vi "NFindBlock.vi"(6 "Start pos":dbl[](array[numeric])=[1161.9163378402552, 774.3453732417895, -2809.9800957108705], 7 "Robot pos":dbl[](array[numeric])=[1630.1539120368434, 560.2708584885918, -4533.599258498874], 9 "Y array":dbl[](array[numeric])=[1951.9460733978328, 2174.013680158977, 2100.374349178618, 2027.3757209543814, 1956.3808654729685, 1887.0818616789568, 1760.9212330614585, 1711.1248280430027, 1665.8553251480664, 1620.1460768722577, 1574.622711636553, 1528.915202610297, 1482.2464785728923, 1343.483778512897, 1271.9279899122423, 1200.9260176050532, 1130.2822245353427, 1056.6497434670005, 977.0249347379225, 894.9824777519775, 813.45928692706, 728.5434146890511, 639.3942546253647, 549.8327407334499, 1303.2154100813484, 1326.243227689847, 1344.7706940544083, 1355.2988665944963, 1366.388334703981, 1376.2633344507678, 1387.3858605477956, 1387.3395311652666, 1396.1291038661302, 1403.8469963592477, 1406.044876812333, 1415.0186919401144, 1397.8349011686557, 1389.429356203805, 1373.0493553890178, 1358.50073650405, 1336.518228027625, 1318.298945741701, 1298.2767133270827, 1269.645856509089, 1247.0060082973419, 1218.7298653868406, 1183.8278258507207, 1145.3413977831867, 1095.4051844135165, 740.1869782093036, 23.99749729169054, 207.57463312261515, 805.7866319591266, 817.4400934673912, 818.5072362633629, 821.8761093260312, 819.8466805765689, 815.5148614886957, 824.0348328052428, 822.83465659537, 464.25266290449787, 585.1972125022019, 673.3405719807987, 766.7834885260188, 829.9570043298224, 884.1159474944076, 942.2369923838124, 996.1391626333278, 1039.3858638370557, 1085.488380279815, 1121.1125501237539, 1158.9307810852838, 1199.0936518769847, 1232.3129831228168, 1262.7377623276616, 1295.8349424882083, 1327.0721507495969, 1351.6669897111408, 1381.610245921101, 1407.2042223079936, 1432.41398094842, 1455.6856235905836, 1480.4306726783261, 1504.798361007342, 1526.2017306501602, 1548.0612165553393, 1569.6740260629588, 1591.7294048725746, 1613.2991676495703, 1634.8604391685087, 1656.4354887780153, 1678.0312036831035, 1699.883503431187, 1721.697021418771, 1744.5419621698122, 1767.0232011908681, 1791.2765152829897, 1814.449222843856, 1839.835232297668, 1863.752486798985, 1893.2873761061576, 1920.0726997144748, 1947.1771574479276, 1977.1918557365602, 2006.6114986258722, 2038.738335023901, 2073.2489083779924], 11 "X array":dbl[](array[numeric])=[1456.236150721847, 2284.533179777942, 2284.295725041913, 2279.991717965582, 2277.559411659486, 2278.1640532747815, 1753.1245409459352, 1716.4389737560573, 1724.7236952758367, 1721.2277238523825, 1718.9409089266371, 1718.8560835426865, 1723.9084271181484, 2274.4657816362965, 2283.4290603719764, 2282.591506521835, 2275.933207563841, 2274.9011301894657, 2284.7297704411108, 2292.7393177141944, 2292.3894714354046, 2292.699070874971, 2294.1694429640193, 2289.556019135518, 1040.5543330524129, 971.0740911191788, 915.9285856561455, 876.5234537267738, 840.7217814934232, 809.8216040555186, 780.8330337957166, 764.060398067916, 741.5121042376231, 721.7303887631895, 707.2373183722646, 689.5683336144892, 687.7576310935447, 680.3237144270757, 676.1209640169212, 670.0595292290169, 665.7321550690846, 658.6348762850175, 650.7889504733546, 643.5411527092657, 633.0560483284596, 621.8034014080613, 609.1996311053018, 594.224150273746, 576.6659280289391, 552.5990468637154, 483.2931255199142, 435.96399945066634, 455.4873314565852, 424.3582060008291, 391.53830766967513, 358.83602127074283, 324.1814884543077, 287.79293769130516, 254.9578550007017, 217.68565770866226, 10.547948949944026, 16.44230453278045, 13.542194258521594, 20.905016219413795, 15.560927519712452, 8.354782022813243, 8.279634233092246, 9.24881034641711, 4.650382600406422, 6.133277633590055, -0.0200408321689686, -1.189523779123516, 3.6713147312194354, 2.6441058297686166, -0.001729572684149782, 4.004890987488247, 7.965285481202459, 1.861479901915235, 8.6812954675475, 8.620211928824281, 9.703950971307904, 7.133609402406625, 11.322817599481725, 17.560083004918255, 13.057057506790496, 11.375796251208232, 8.576030352070497, 11.61472095873304, 10.529175885171588, 14.291144028101057, 11.900291514034304, 12.358671231711238, 11.684690157692211, 12.872594767662067, 10.03511447810198, 11.068894101653681, 7.264975406698252, 9.275179363476706, 6.6484746079565, 9.784068575249455, 2.1939999046841003, 3.1971680745385944, 5.458041523244977, 4.762383636342437, 7.242210496859455, 7.977667065473892, 8.065439991600666]) -> (0 "Group Lidar Map":cluster{dbl[], dbl[]}[](graph)=[{[], []}, {[1760.9212330614585, 1482.2464785728923], [1716.4389737560573, 1716.4389737560573]}, {[], []}, {[], []}, {[], []}, {[824.0348328052428, 824.0348328052428], [455.4873314565852, 217.68565770866226]}], 2 "Line Array":dbl[][][](array[numeric])=[[[0.0, 0.0], [0.0, 0.0], [0.0, 0.0]], [[1716.4389737560573, 1716.4389737560573], [1760.9212330614585, 1482.2464785728923], [1.5, 1.5]], [[0.0, 0.0], [0.0, 0.0], [0.0, 0.0]], [[0.0, 0.0], [0.0, 0.0], [0.0, 0.0]], [[0.0, 0.0], [0.0, 0.0], [0.0, 0.0]], [[455.4873314565852, 217.68565770866226], [824.0348328052428, 824.0348328052428], [0.0, 0.0]]], 3 "Empty Array":dbl[][][](array[numeric]))   [LabVIEW 2018]
panel:
  out "Array X1":dbl[](array[numeric])=[0.0, 36.68556718987793, 463.88840502347375, 0.0, 0.0, 237.80167374792293]
  out "Array Y1":dbl[](array[numeric])=[0.0, 278.6747544885661, 319.6135075265979, 0.0, 0.0, 18.24820084611622]
  out "Array Y":dbl[][](array[numeric])=[[1951.9460733978328, 0.0, 0.0, 0.0, 0.0, 0.0, 0.0, 0.0, 0.0, 0.0, 0.0, 0.0, 0.0, 0.0, 0.0, 0.0, 0.0, 0.0, 0.0, 0.0, 0.0, 0.0, 0.0, 0.0, 0.0], [1760.9212330614585, 1711.1248280430027, 1665.8553251480664, 1620.1460768722577, 1574.622711636553, 1528.915202610297, 1482.2464785728923, 0.0, 0.0, 0.0, 0.0, 0.0, 0.0, 0.0, 0.0, 0.0, 0.0, 0.0, 0.0, 0.0, 0.0, 0.0, 0.0, 0.0, 0.0], [1303.2154100813484, 1326.243227689847, 1344.7706940544083, 1355.2988665944963, 1366.388334703981, 1376.2633344507678, 1387.3858605477956, 1387.3395311652666, 1396.1291038661302, 1403.8469963592477, 1406.044876812333, 1415.0186919401144, 1397.8349011686557, 1389.429356203805, 1373.0493553890178, 1358.50073650405, 1336.518228027625, 1318.298945741701, 1298.2767133270827, 1269.645856509089, 1247.0060082973419, 1218.7298653868406, 1183.8278258507207, 1145.3413977831867, 1095.4051844135165], [740.1869782093036, 0.0, 0.0, 0.0, 0.0, 0.0, 0.0, 0.0, 0.0, 0.0, 0.0, 0.0, 0.0, 0.0, 0.0, 0.0, 0.0, 0.0, 0.0, 0.0, 0.0, 0.0, 0.0, 0.0, 0.0], [207.57463312261515, 0.0, 0.0, 0.0, 0.0, 0.0, 0.0, 0.0, 0.0, 0.0, 0.0, 0.0, 0.0, 0.0, 0.0, 0.0, 0.0, 0.0, 0.0, 0.0, 0.0, 0.0, 0.0, 0.0, 0.0], [805.7866319591266, 817.4400934673912, 818.5072362633629, 821.8761093260312, 819.8466805765689, 815.5148614886957, 824.0348328052428, 822.83465659537, 0.0, 0.0, 0.0, 0.0, 0.0, 0.0, 0.0, 0.0, 0.0, 0.0, 0.0, 0.0, 0.0, 0.0, 0.0, 0.0, 0.0]]
  out "Array X":dbl[][](array[numeric])=[[1456.236150721847, 0.0, 0.0, 0.0, 0.0, 0.0, 0.0, 0.0, 0.0, 0.0, 0.0, 0.0, 0.0, 0.0, 0.0, 0.0, 0.0, 0.0, 0.0, 0.0, 0.0, 0.0, 0.0, 0.0, 0.0], [1753.1245409459352, 1716.4389737560573, 1724.7236952758367, 1721.2277238523825, 1718.9409089266371, 1718.8560835426865, 1723.9084271181484, 0.0, 0.0, 0.0, 0.0, 0.0, 0.0, 0.0, 0.0, 0.0, 0.0, 0.0, 0.0, 0.0, 0.0, 0.0, 0.0, 0.0, 0.0], [1040.5543330524129, 971.0740911191788, 915.9285856561455, 876.5234537267738, 840.7217814934232, 809.8216040555186, 780.8330337957166, 764.060398067916, 741.5121042376231, 721.7303887631895, 707.2373183722646, 689.5683336144892, 687.7576310935447, 680.3237144270757, 676.1209640169212, 670.0595292290169, 665.7321550690846, 658.6348762850175, 650.7889504733546, 643.5411527092657, 633.0560483284596, 621.8034014080613, 609.1996311053018, 594.224150273746, 576.6659280289391], [552.5990468637154, 0.0, 0.0, 0.0, 0.0, 0.0, 0.0, 0.0, 0.0, 0.0, 0.0, 0.0, 0.0, 0.0, 0.0, 0.0, 0.0, 0.0, 0.0, 0.0, 0.0, 0.0, 0.0, 0.0, 0.0], [435.96399945066634, 0.0, 0.0, 0.0, 0.0, 0.0, 0.0, 0.0, 0.0, 0.0, 0.0, 0.0, 0.0, 0.0, 0.0, 0.0, 0.0, 0.0, 0.0, 0.0, 0.0, 0.0, 0.0, 0.0, 0.0], [455.4873314565852, 424.3582060008291, 391.53830766967513, 358.83602127074283, 324.1814884543077, 287.79293769130516, 254.9578550007017, 217.68565770866226, 0.0, 0.0, 0.0, 0.0, 0.0, 0.0, 0.0, 0.0, 0.0, 0.0, 0.0, 0.0, 0.0, 0.0, 0.0, 0.0, 0.0]]
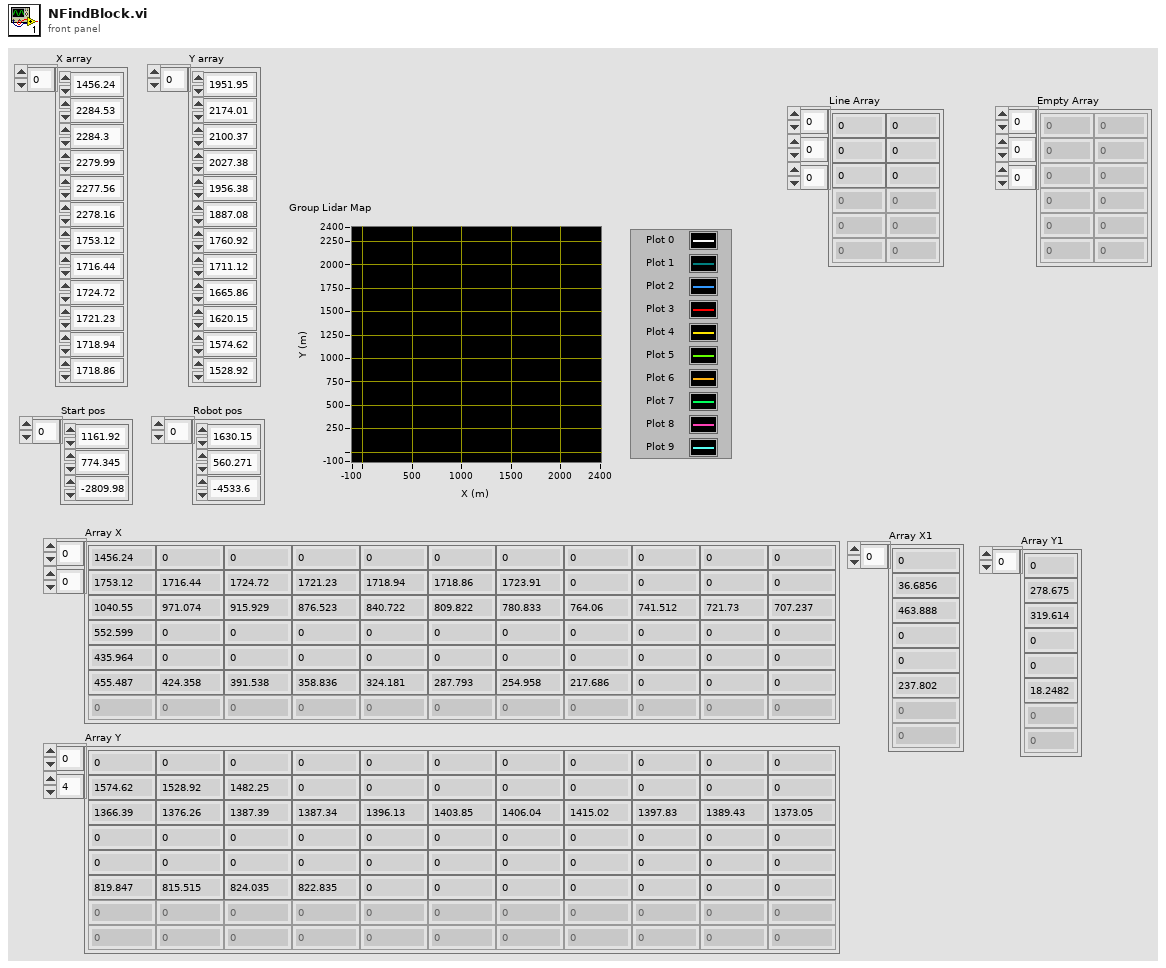
[diagram p1: front panel]
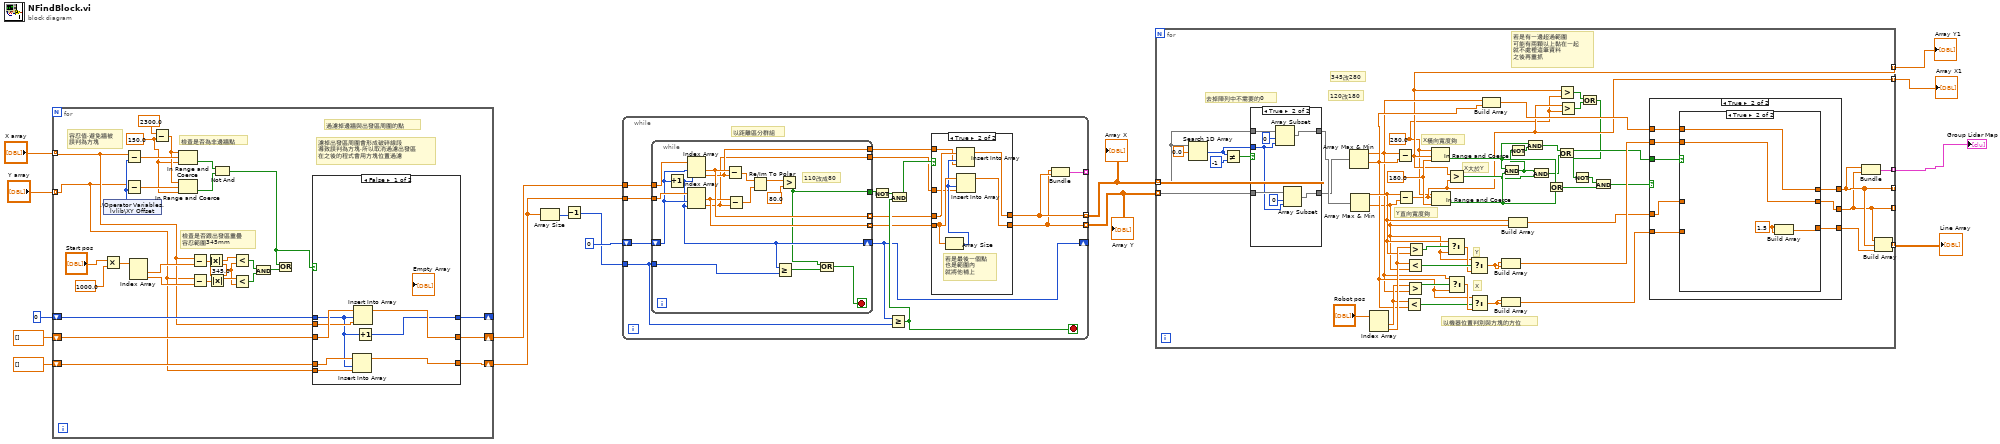
[diagram p0: block diagram]
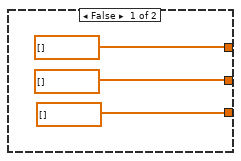
[diagram p3: hidden frame]
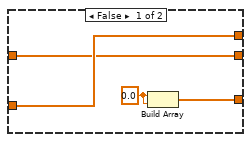
[diagram p4: hidden frame]
diagram:
  n1 = for {
    tunnel: "X array" -> [w23] mode=indexing
    tunnel: "Y array" -> [w22] mode=indexing
    shift-right: [w21] -> w11
    shift-left: dbl[] [] -> [w26]
    shift-right: [w20] -> w9
    shift-left: dbl[] [] -> [w25]
    shift-right: [w19] -> _
    shift-left: 0 -> [w24]
    w34 = 345.0
    w41 = 150.0 ("y")
    # "容忍值,避免牆被\n誤判為方塊"
    # "濾掉出發區周圍會形成破碎線段\n導致誤判為方塊,所以取消過濾出發區\n在之後的程式會用方塊位置過濾"
    # "過濾掉邊牆與出發區周圍的點"
    # "檢查是否為非邊牆點"
    # "檢查是否跟出發區重疊\n容忍範圍345mm"
    n2 = shared-variable ".\\Operator Variables.lvlib\\XY Offset"() -> (w46:i16)  [unwired: 1 in, 1 out]
    n3 = Multiply(x="Start pos", y=1000.0) -> (x*y=w33:dbl[])
    n4 = Subtract(x=w23, y=w46) -> (x-y=w45:dbl)
    n5 = Subtract(x=w22, y=w46) -> (x-y=w44:dbl)
    n6 = Index Array(array=w33) -> (element #1=w36:dbl, element #2=w35:dbl)  [unwired: 2 in]
    n7 = Subtract(x=2300.0 ("upper limit"), y=w41) -> (x-y=w42:dbl)
    n8 = In Range and Coerce(upper limit=w42, x=w45, lower limit=w41) -> (In Range?=w28:bool)  [unwired: 1 out]
    n9 = In Range and Coerce(upper limit=w42, x=w44, lower limit=w41) -> (In Range?=w27:bool)  [unwired: 1 out]
    n10 = Subtract(x=w23, y=w36) -> (x-y=w37:dbl)
    n11 = Subtract(x=w22, y=w35) -> (x-y=w38:dbl)
    n12 = Absolute Value(x=w37) -> (abs(x)=w39:dbl)
    n13 = Absolute Value(x=w38) -> (abs(x)=w40:dbl)
    n14 = Not And(1:w27, 2:w28) -> (0:w17:bool)
    n15 = Less?(x=w39, y=w34) -> (x < y?=w30:bool)
    n16 = Less?(x=w40, y=w34) -> (x < y?=w29:bool)
    n17 = And(x=w30, y=w29) -> (x .and. y?=w18:bool)
    n18 = Or(x=w17, y=w18) -> ()  [unwired: 1 out]
    n19 = case shown="False" w17 {
      tunnel: w26 -> [w54 w56]
      tunnel: w25 -> [w53 w55]
      tunnel: w24 -> [w51 w57]
      tunnel: w23 -> [w52 _]
      tunnel: w22 -> [w50 _]
      tunnel: [w49 w56] -> w21
      tunnel: [w48 w55] -> w20
      tunnel: [w47 w57] -> w19
      frame False {
        n20 = Insert Into Array(array=w53, index=w51, new element=w50) -> (w48:dbl[])
        n21 = Insert Into Array(array=w54, index=w51, new element=w52) -> (w49:dbl[])
        n22 = Increment(x=w51) -> (x+1=w47:i32)
      }
      frame True {
      }
    }
  }
  n23 = Array Size(array=w9) -> (size(s)=w8:i32)
  n24 = Decrement(x=w8) -> (x-1=w7:i32)
  n25 = while {
    tunnel: w11 -> [w73]
    tunnel: w9 -> [w71]
    tunnel: w7 -> [w70]
    shift-right: [w60] -> _
    shift-left: 0 -> [w72]
    tunnel: [w62] -> w6 mode=indexing
    tunnel: [w61] -> w5 mode=indexing
    tunnel: [w69] -> _ mode=indexing
    stop <- w66 stop-if-true
    # "以距離區分群組"
    n26 = while {
      tunnel: w73 -> [w98]
      tunnel: w71 -> [w97]
      shift-right: [w91] -> w60
      shift-left: w72 -> [w96]
      tunnel: w70 -> [w90]
      tunnel: [w87] -> w64 mode=indexing
      tunnel: [w86] -> w63 mode=indexing
      tunnel: [w85] -> w68
      tunnel: [w84] -> w59
      tunnel: [w83] -> w58
      stop <- w88 stop-if-true
      # "110改成80"
      n27 = Increment(x=w96) -> (x+1=w91:i32)
      n28 = Index Array(array=w98, index #1=w96, index #2=w91) -> (element #1=w87:dbl, element #2=w84:dbl)
      n29 = Index Array(array=w97, index #1=w96, index #2=w91) -> (element #1=w86:dbl, element #2=w83:dbl)
      n30 = Subtract(x=w87, y=w84) -> (x-y=w95:dbl)
      n31 = Subtract(x=w86, y=w83) -> (x-y=w94:dbl)
      n32 = Re/Im To Polar(2:w94, 3:w95) -> (1:w93:dbl)  [unwired: 1 out]
      n33 = Greater Or Equal?(x=w91, y=w90) -> (x >= y?=w89:bool)
      n34 = Greater?(x=w93, y=80.0) -> (0:w85:bool)
      n35 = Or(x=w85, y=w89) -> (x .or. y?=w88:bool)
    }
    n36 = Not(x=w68) -> (.not. x?=w67:bool)
    n37 = Greater Or Equal?(x=w60, y=w70) -> (x >= y?=w66:bool)
    n38 = And(x=w67, y=w66) -> (x .and. y?=w65:bool)
    n39 = case shown="True" w65 {
      tunnel: w64 -> [w75 w82]
      tunnel: w63 -> [w74 w81]
      tunnel: [w75 w77] -> w62
      tunnel: [w74 w76] -> w61
      tunnel: w59 -> [_ w79]
      tunnel: w58 -> [_ w78]
      frame False {
      }
      frame True {
        # "若是最後一個點\n也是範圍內\n就將他補上"
        n40 = Array Size(array=w81) -> (size(s)=w80:i32)
        n41 = Insert Into Array(array=w82, index=w80, new element=w79) -> (w77:dbl[])
        n42 = Insert Into Array(array=w81, index=w80, new element=w78) -> (w76:dbl[])
      }
    }
    n43 = Bundle(w61, w62) -> (w69:cluster{dbl[], dbl[]})  [unwired: 1 in]
  }
  "Array X" <- w6
  "Array Y" <- w5
  n44 = for {
    tunnel: w6 -> [w124] mode=indexing
    tunnel: w5 -> [w122] mode=indexing
    tunnel: [w113] -> _ mode=indexing
    tunnel: [w112] -> _ mode=indexing
    tunnel: [w128] -> w3 mode=indexing
    tunnel: [w120] -> w4 mode=indexing
    tunnel: [w107] -> w2 mode=indexing
    tunnel: [w106] -> w1 mode=indexing
    w105 = 280.0 ("lower limit")
    w148 = 180.0 ("lower limit")
    # "若是有一邊超過範圍\n可能有兩顆以上黏在一起\n就不處裡這筆資料\n之後再重抓"
    # "120改180"
    # "345改280"
    # "X大於Y"
    # "去掉陣列中不需要的0"
    # "以機器位置判別與方塊的方位"
    # "Y直向寬度夠"
    # "X橫向寬度夠"
    # "X"
    # "Y"
    n45 = Search 1D Array(1D array=w124, element=0.0) -> (index of element=w123:i32)  [unwired: 1 in]
    n46 = Not Equal?(x=w123, y=-1) -> (x != y?=w125:bool)
    n47 = case shown="True" w125 {
      tunnel: w124 -> [w150 w157]
      tunnel: [w150 w155] -> w119
      tunnel: w123 -> [_ w151]
      tunnel: w122 -> [w149 w153]
      tunnel: [w149 w152] -> w118
      frame False {
      }
      frame True {
        n48 = Array Subset(array=w157, index=0, length=w151) -> (w155:dbl[])
        n49 = Array Subset(array=w153, index=0, length=w151) -> (w152:dbl[])
      }
    }
    n50 = Array Max & Min(array=w118) -> (max value=w111:dbl, min value=w114:dbl)  [unwired: 2 out]
    n51 = Array Max & Min(array=w119) -> (max value=w117:dbl, min value=w109:dbl)  [unwired: 2 out]
    n52 = Index Array(array="Robot pos") -> (element #1=w145:dbl, element #2=w146:dbl)  [unwired: 2 in]
    n53 = Subtract(x=w111, y=w114) -> (x-y=w107:dbl)
    n54 = Subtract(x=w117, y=w109) -> (x-y=w106:dbl)
    n55 = Less?(x=w145, y=w114) -> (x < y?=w141:bool)
    n56 = Less?(x=w146, y=w109) -> (x < y?=w144:bool)
    n57 = Greater?(x=w145, y=w111) -> (0:w115:bool)
    n58 = Greater?(x=w146, y=w117) -> (0:w116:bool)
    n59 = In Range and Coerce(upper limit=w105, x=w107, lower limit=w148) -> (In Range?=w134:bool)  [unwired: 1 out]
    n60 = In Range and Coerce(upper limit=w105, x=w106, lower limit=w148) -> (In Range?=w136:bool)  [unwired: 1 out]
    n61 = Select(t=w117, s=w116, f=w109) -> (s? t:f=w143:dbl)
    n62 = Greater?(x=w107, y=w106) -> (0:w135:bool)
    n63 = Select(t=w111, s=w115, f=w114) -> (s? t:f=w142:dbl)
    n64 = Select(t=w109, s=w144, f=w143) -> (s? t:f=w140:dbl)
    n65 = Select(t=w114, s=w141, f=w142) -> (s? t:f=w139:dbl)
    n66 = Build Array(w111, w114) -> (w110:dbl[])
    n67 = Build Array(w140, w140) -> (w138:dbl[])
    n68 = Build Array(w139, w139) -> (w137:dbl[])
    n69 = And(x=w134, y=w136) -> (x .and. y?=w132:bool)
    n70 = Build Array(w117, w109) -> (w108:dbl[])
    n71 = Not(x=w132) -> (.not. x?=w133:bool)
    n72 = And(x=w134, y=w133) -> (x .and. y?=w131:bool)
    n73 = And(x=w132, y=w135) -> (x .and. y?=w130:bool)
    n74 = Or(x=w134, y=w136) -> (x .or. y?=w102:bool)
    n75 = Or(x=w131, y=w130) -> (x .or. y?=w129:bool)
    n76 = Greater?(x=w107, y=w105) -> (0:w104:bool)
    n77 = Greater?(x=w106, y=w105) -> (0:w103:bool)
    n78 = Or(x=w104, y=w103) -> (x .or. y?=w99:bool)
    n79 = Not(x=w99) -> (.not. x?=w100:bool)
    n80 = And(x=w100, y=w102) -> (x .and. y?=w101:bool)
    n81 = case shown="True" w101 {
      tunnel: w110 -> [_ w166]
      tunnel: w108 -> [_ w162]
      tunnel: w138 -> [_ w164]
      tunnel: w137 -> [_ w163]
      tunnel: [dbl[] [] w167] -> w113
      tunnel: [dbl[] [] w165] -> w112
      tunnel: w129 -> [_ w168]
      tunnel: [dbl[] [] w161] -> w121
      frame False {
      }
      frame True {
        n82 = case shown="True" w168 {
          tunnel: [w172 w176] -> w167
          tunnel: w166 -> [_ w176]
          tunnel: [w171 w175] -> w165
          tunnel: w164 -> [_ w175]
          tunnel: w163 -> [w172 _]
          tunnel: w162 -> [w171 _]
          tunnel: [w169 w173] -> w161
          frame False {
            w170 = 0.0 ("element")
            n83 = Build Array(w170, w170) -> (w169:dbl[])
          }
          frame True {
            w174 = 1.5 ("element")
            n84 = Build Array(w174, w174) -> (w173:dbl[])
          }
        }
      }
    }
    n85 = Bundle(w113, w112) -> (w128:cluster{dbl[], dbl[]})  [unwired: 1 in]
    n86 = Build Array(w112, w113, w121) -> (w120:dbl[][])
  }
  "Group Lidar Map" <- w3
  "Line Array" <- w4
  "Array Y1" <- w2
  "Array X1" <- w1
